vi "turretPitchLogical.vi"() -> ()   [LabVIEW 2016]
uses:
  <vilib>/Rock Robotics/WPI/PWM/Servo/WPI_ServoDeviceRef.ctl
  <vilib>/Rock Robotics/SystemInterfaces/DIO/FPGA_DIOPWMChannel.ctl
  <vilib>/Rock Robotics/WPI/PWM/WPI_PWMDeadband.ctl
  <vilib>/addons/control/pid/pid.llb/PID (DBL).vi
  <vilib>/addons/control/pid/NI_PID_pid.lvlib
panel:
  out "s? t:f":dbl
  in  "range":cluster{"high":dbl, "low":dbl}
  in  "softstop":dbl
  in  "desiredAngle":dbl format="%.2f"
  in  "currentAngle":dbl format="%.2f"
  in  "output range":cluster{"output high":dbl, "output low":dbl}={"output high"=100.0, "output low"=-100.0} {"output low" format="%.2f"; "output high" format="%.2f"}
  in  "PID gains":T1={"proportional gain (Kc)"=1.0, "integral time (Ti, min)"=0.01, "derivative time (Td, min)"=0.0} {"derivative time (Td, min)" format="%.3f"; "integral time (Ti, min)" format="%.3f"; "proportional gain (Kc)" format="%.3f"}
  in  "servoPitchDevRef":T2={"DeviceStatus"={"status"=FALSE, "code"=0, "source"=""}, "PWM Channel"=enum."Invalid", "DeadBand"={"Name"="", "maxPositivePwm"=0, "minPositivePwm"=0, "centerPwm"=0, "maxNegativePwm"=0, "minNegativePwm"=0, "angularRange"=0}}
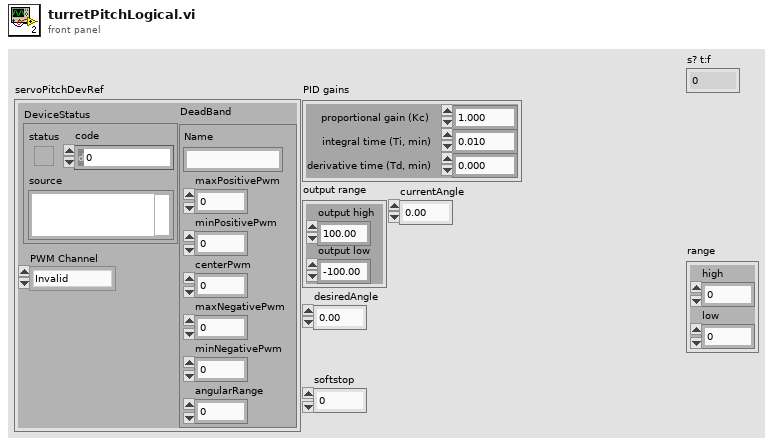
[diagram p1: front panel]
types:
  T1 = cluster{"proportional gain (Kc)":dbl, "integral time (Ti, min)":dbl, "derivative time (Td, min)":dbl}
  T2 = typedef "WPI_ServoDeviceRef.ctl" = cluster{"DeviceStatus":errorcluster, "PWM Channel":T3, "DeadBand":T4}
  T3 = typedef "FPGA_DIOPWMChannel.ctl" = enum8{"PWM 0", "PWM 1", "PWM 2", "PWM 3", "PWM 4", "PWM 5", "PWM 6", "PWM 7", "PWM 8", "PWM 9", "PWM MXP 0", "PWM MXP 1", "PWM MXP 2", "PWM MXP 3", "PWM MXP 4", "PWM MXP 5", "PWM MXP 6", "PWM MXP 7", "PWM MXP 8", "PWM MXP 9", "Invalid"}
  T4 = typedef "WPI_PWMDeadband.ctl" = cluster{"Name":string, "maxPositivePwm":i32, "minPositivePwm":i32, "centerPwm":i32, "maxNegativePwm":i32, "minNegativePwm":i32, "angularRange":u16}
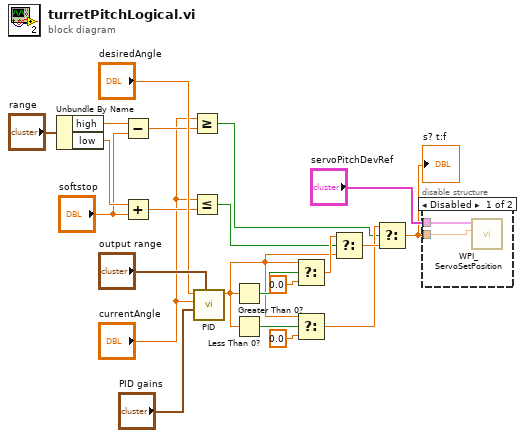
[diagram p0: block diagram]
diagram:
  n1 = Unbundle By Name("range") -> ("high"=w11:dbl, "low"=w10:dbl)
  n2 = Subtract(x=w11, y="softstop") -> (x-y=w5:dbl)
  n3 = Add(x=w10, y="softstop") -> (x+y=w3:dbl)
  n4 = Greater Or Equal?(x="currentAngle", y=w5) -> (x >= y?=w4:bool)
  n5 = Less Or Equal?(x="currentAngle", y=w3) -> (x <= y?=w1:bool)
  n6 = call-poly <vilib>:"PID.vi"("output range"="output range", "PID gains"="PID gains", "process variable"="currentAngle", "setpoint"="desiredAngle") -> ("output"=w6:dbl)  [unwired: 6 in, 1 out]
  n7 = Greater Than 0?(x=w6) -> (x > 0?=w7:bool)
  n8 = Less Than 0?(x=w6) -> (x < 0?=w8:bool)
  n9 = Select(t=w6, s=w7, f=0.0) -> (s? t:f=w14:dbl)
  n10 = Select(t=w6, s=w8, f=0.0) -> (s? t:f=w15:dbl)
  n11 = Select(t=w14, s=w1, f=w6) -> (s? t:f=w16:dbl)
  n12 = Select(t=w15, s=w4, f=w16) -> (s? t:f=w17:dbl)
  "s? t:f" <- w17
  n13 = disable-structure shown="Disabled" {
    disable-tunnel: "servoPitchDevRef" -> [w24 _]
    disable-tunnel: w17 -> [w23 _]
    frame Disabled {
      n14 = call <vilib>:"WPI_ServoSetPosition.vi"("Position"=w23, "ServoDeviceRef"=w24) -> ()  [unwired: 8 in, 2 out]
    }
    frame Enabled {
    }
  }
